vi "saveProject.vi"(8 "error in (no error)":errorcluster, 11 "VGS_RemoteControlClient in":refnum<class "VGS_RemoteControlClient.lvclass">) -> (0 "error out":errorcluster, 3 "VGS_RemoteControlClient out":refnum<class "VGS_RemoteControlClient.lvclass">)   [LabVIEW 2022 SP3, in "LV_VGS.lvlib" / "VGS_RemoteControlClient.lvclass"]
doc: "<B>Saves the last changes of a loaded VG Project. </B>\n\nParameters\nhandle A valid remote handle. \nprojectName The absolute path to a VG project. \n\nEmit error RemoteControlServiceIsNotAvailableException if the remote control service doesn't run. \nEmit error GenericRemoteControlErrorException if an internal error occurs. \nEmit error InvalidRemoteHandleException if the remote handle is not valid."
uses:
  VGS_RemoteControlClient.lvclass
  VGS_RemoteControlClient.lvclass/VGS_RemoteControlClient.ctl
  C:/Users/Andrey/Desktop/hajo/LV_VGS/vgs_project.dll
  vgs_project.dll
panel:
  in  "projectName":string
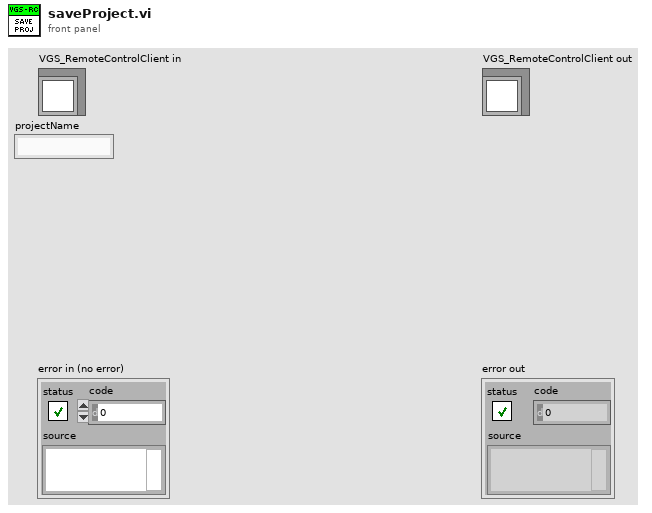
[diagram p1: front panel]
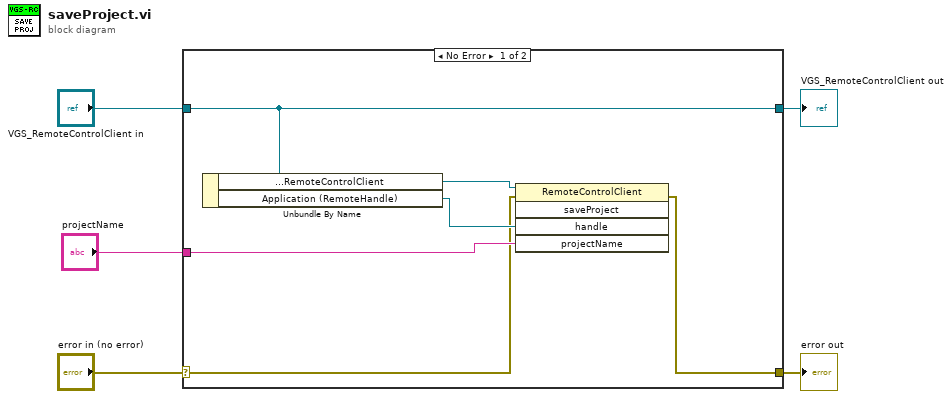
[diagram p0: block diagram]
diagram:
  n1 = case shown="No Error" "error in (no error)" {
    selector: "error in (no error)" -> [w7 w13]
    tunnel: [w6 w13] -> w4
    tunnel: [w11 w12] -> w2
    tunnel: "VGS_RemoteControlClient in" -> [w11 w12]
    tunnel: "projectName" -> [w8 _]
    frame No Error {
      n2 = Unbundle By Name(w11) -> ("VGS.Project.Interop.RemoteControlClient"=w10:refnum<k24>, "Application (RemoteHandle)"=w9:refnum<k24>)
      n3 = invoke class="RemoteControlClient" method="saveProject"(reference=w10, error in=w7, "handle"=w9, "projectName"=w8) -> (error out=w6:errorcluster)  [unwired: 1 in, 4 out]
    }
    frame Error {
    }
  }
  "error out" <- w4
  "VGS_RemoteControlClient out" <- w2
